vi "Control Panel Values Changed.vi"(8 "error in (no error)":errorcluster, 9 "Old value":variant, 10 "New value":variant, 11 "LakeShore 335 in":refnum<class "LakeShore 335.lvclass">) -> (0 "error out":errorcluster, 3 "LakeShore 335 out":refnum<class "LakeShore 335.lvclass">)   [LabVIEW 2015, in "LakeShore 335.lvclass"]
uses:
  LakeShore 335.lvclass
  LakeShore335 Front Panel Data.ctl
  LakeShore335 Heater Ranges.ctl
  Neocera/Neocera Set Point Aproach.ctl
  Instrument/Read VISA Resource.vi
  Instrument/Write VISA Resource.vi
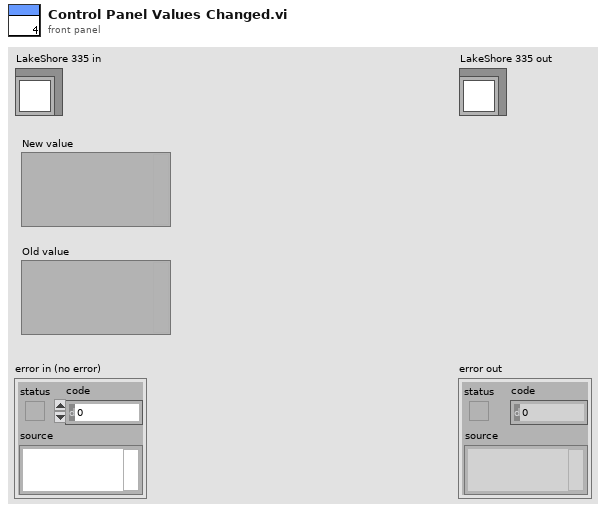
[diagram p1: front panel]
types:
  T1 = typedef "LakeShore335 Front Panel Data.ctl" = cluster{"Heater":bool, "A":bool, "B":bool, " RAW":bool, "Set point":dbl, "Set Heater Range":T2, "Approach":T3, "Ramp rate, K/min":dbl}
  T2 = typedef "LakeShore335 Heater Ranges.ctl" = enum16{"0 (Off)", "1 Low", "2 Medium", "3 High"}
  T3 = typedef "Neocera Set Point Aproach.ctl" = enum16{"Instant", "Ramp"}
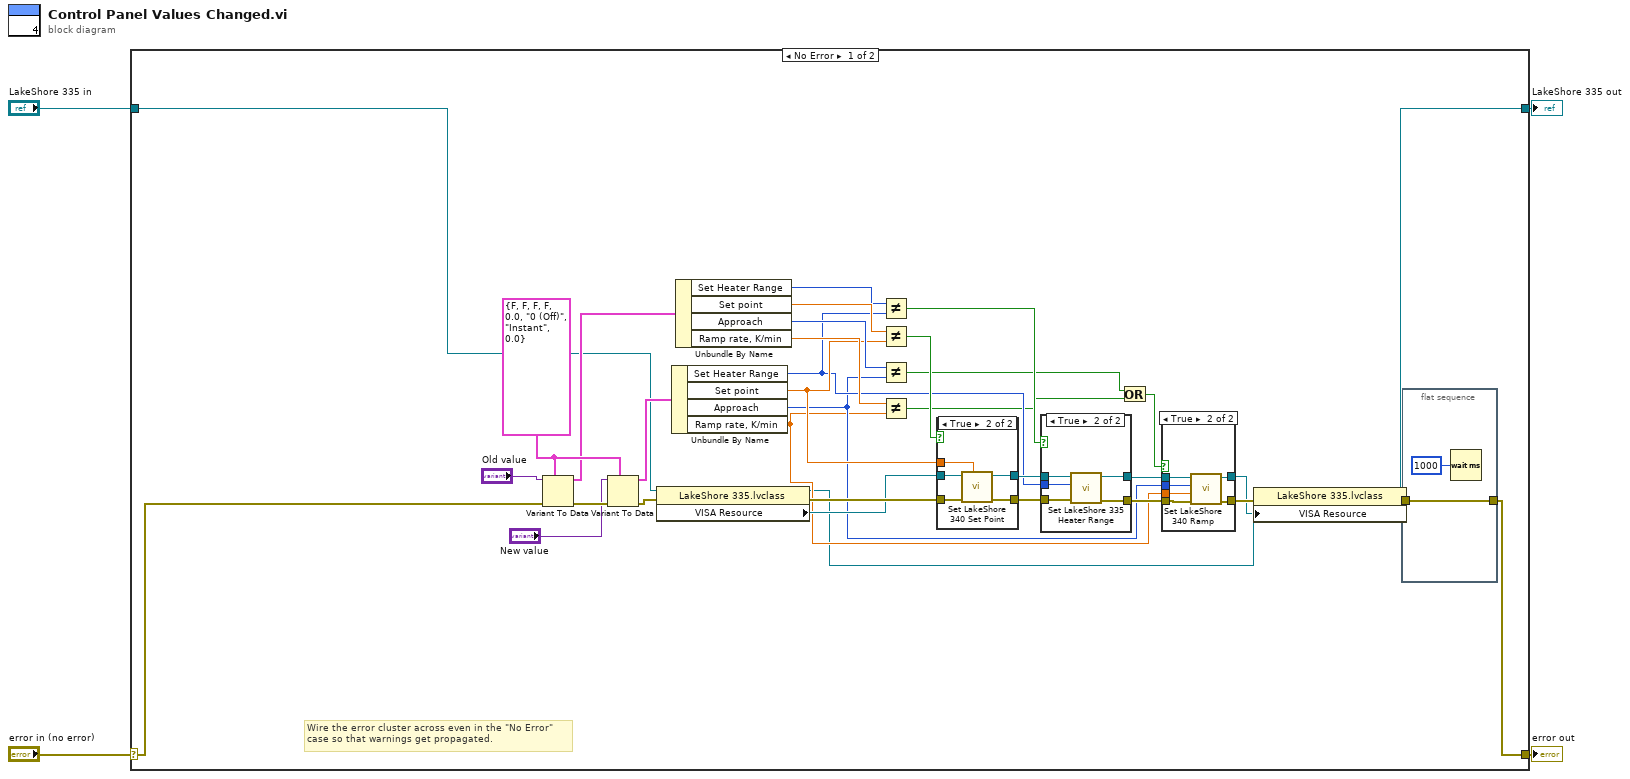
[diagram p0: block diagram]
diagram:
  n1 = case shown="No Error" "error in (no error)" {
    selector: "error in (no error)" -> [w9 w64]
    tunnel: [w5 w64] -> w3
    tunnel: [w7 w63] -> w1
    tunnel: "LakeShore 335 in" -> [w8 w63]
    frame No Error {
      w34 = T1 {"Heater"=FALSE, "A"=FALSE, "B"=FALSE, " RAW"=FALSE, "Set point"=0.0, "Set Heater Range"=enum."0 (Off)", "Approach"=enum."Instant", "Ramp rate, K/min"=0.0} ("Data")
      # "Wire the error cluster across even in the \"No Error\"\ncase so that warnings get propagated."
      n2 = Variant To Data(error in=w9, type=w34, Variant="Old value") -> (data=w29:T1, error out=w38:errorcluster)
      n3 = Variant To Data(error in=w38, type=w34, Variant="New value") -> (data=w28:T1, error out=w37:errorcluster)
      n4 = property class="LakeShore 335.lvclass"(reference=w8, error in=w37) -> (reference out=w11:refnum<class "LakeShore 335.lvclass">, error out=w27:errorcluster, "VISA Resource"=w26:refnum<visa-resource-name>)
      n5 = Unbundle By Name(w28) -> ("Set Heater Range"=w21:T2, "Set point"=w24:dbl, "Approach"=w14:T3, "Ramp rate, K/min"=w13:dbl)
      n6 = Unbundle By Name(w29) -> ("Set Heater Range"=w32:T2, "Set point"=w33:dbl, "Approach"=w31:T3, "Ramp rate, K/min"=w30:dbl)
      n7 = Not Equal?(x=w32, y=w21) -> (x != y?=w20:bool)
      n8 = Not Equal?(x=w33, y=w24) -> (x != y?=w25:bool)
      n9 = Not Equal?(x=w31, y=w14) -> (x != y?=w18:bool)
      n10 = Not Equal?(x=w30, y=w13) -> (x != y?=w17:bool)
      n11 = case shown="True" w25 {
        tunnel: w27 -> [w57 w62]
        tunnel: w26 -> [w56 w61]
        tunnel: w24 -> [_ w60]
        tunnel: [w57 w59] -> w23
        tunnel: [w56 w58] -> w22
        frame False {
        }
        frame True {
          n12 = call "Set LakeShore 340 Set Point.vi"("Set point"=w60, "error in (no error)"=w62, "VISA Resource Name"=w61) -> ("error out"=w59:errorcluster, "VISA Resource Name Out"=w58:refnum<visa-resource-name>)  [unwired: 7 in]
        }
      }
      n13 = case shown="True" w20 {
        tunnel: w23 -> [w50 w55]
        tunnel: w22 -> [w49 w54]
        tunnel: w21 -> [_ w53]
        tunnel: [w49 w52] -> w15
        tunnel: [w50 w51] -> w19
        frame False {
        }
        frame True {
          n14 = call "Set LakeShore 335 Heater Range.vi"("error in (no error)"=w55, "Set Heater Range"=w53, "VISA resource name"=w54) -> ("error out"=w51:errorcluster, "VISA resource name out"=w52:refnum<visa-resource-name>)  [unwired: 7 in]
        }
      }
      n15 = Or(x=w18, y=w17) -> (x .or. y?=w16:bool)
      n16 = case shown="True" w16 {
        tunnel: w19 -> [w42 w48]
        tunnel: w15 -> [w41 w47]
        tunnel: [w42 w45] -> w12
        tunnel: [w41 w46] -> w10
        tunnel: w14 -> [_ w44]
        tunnel: w13 -> [_ w43]
        frame False {
        }
        frame True {
          n17 = call "Set LakeShore 340 Ramp.vi"("error in (no error)"=w48, "Ramp rate, K/min"=w43, "Approach"=w44, "VISA resource name"=w47) -> ("error out"=w45:errorcluster, "VISA resource name out"=w46:refnum<visa-resource-name>)  [unwired: 6 in]
        }
      }
      n18 = property class="LakeShore 335.lvclass"(reference=w11, error in=w12, "VISA Resource"=w10) -> (reference out=w7:refnum<class "LakeShore 335.lvclass">, error out=w6:errorcluster)
      n19 = flat-sequence {
        tunnel: w6 -> [w40]
        tunnel: [w40] -> w5
        frame #0 {
          n20 = Wait (ms)(milliseconds to wait=u32 1000) -> ()  [unwired: 1 out]
        }
      }
    }
    frame Error {
    }
  }
  "error out" <- w3
  "LakeShore 335 out" <- w1
